vi "Read Available HWplugins.vi"(8 "error in (no error)":errorcluster, 11 "Controller in":refnum<class "Controller.lvclass">) -> (0 "error out":errorcluster, 1 "Array of HWplugin Objs":refnum<class "Hardware.lvclass">[](array[class]), 2 "HWplugin Names":string[](array[string]), 3 "Controller out":refnum<class "Controller.lvclass">)   [LabVIEW 2016, in "Controller Actor.lvlib" / "Controller.lvclass"]
uses:
  <userlib>/Common Components/Controller/Controller.lvclass
  <userlib>/Common Components/Hardware/Abstract Hardware/Hardware.lvclass
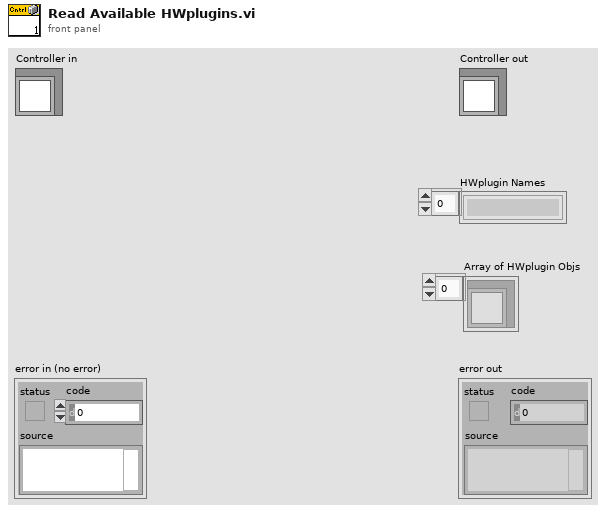
[diagram p1: front panel]
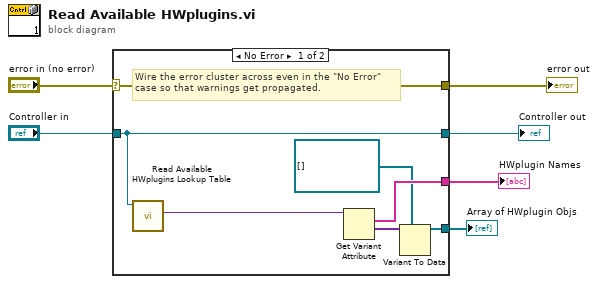
[diagram p0: block diagram]
diagram:
  n1 = case shown="No Error" "error in (no error)" {
    selector: "error in (no error)" -> [w13 w15]
    tunnel: [w13 w15] -> w5
    tunnel: [w12 w14] -> w3
    tunnel: "Controller in" -> [w12 w14]
    tunnel: [w10 _] -> w2
    tunnel: [w7 _] -> w1
    frame No Error {
      # "Wire the error cluster across even in the \"No Error\"\ncase so that warnings get propagated."
      n2 = call <userlib>:"Read Available HWplugins Lookup Table.vi"("Controller in"=w12) -> ("Available HWplugins Lookup Table"=w11:variant)  [unwired: 8 in, 2 out]
      n3 = Get Variant Attribute(Variant=w11) -> (names=w10:string[], values=w9:variant[])  [unwired: 3 in, 2 out]
      n4 = Variant To Data(type=refnum<class "Hardware.lvclass">[] [], Variant=w9) -> (data=w7:refnum<class "Hardware.lvclass">[])  [unwired: 1 in, 1 out]
    }
    frame Error {
    }
  }
  "error out" <- w5
  "Controller out" <- w3
  "HWplugin Names" <- w2
  "Array of HWplugin Objs" <- w1
